vi "FGGA Linelock Settings Procedures.vi"() -> ()   [LabVIEW 2014]
panel:
  out "CO preflight Des 4":string="This issue can be fixed without opening the instrument. However, it may take a little bit of trial an error to get the exact adjustment. The goal is to bring the laser peaks back to their “normal” positions.\n\n1) On the instrument interface, click the Setup button in right hand corner of dashboard\n2) Click Service\n3) In the dialog window, enter ICOService (case sensitive)\n4) Click OK\n5) When the desktop appears, right click anywhere on the desktop\n6) Highlight Open New Window\n7) Click Up twice\n8) Scroll down to folder titled usr\n9) Double click usr\n10)Double click folder titled icos\n11)Double click folder titled conf\n12)Double Click folder titled fgga_ini\n13) If it is the Methane/H2O laser that needs adjusting, right click on filename linelock_0.ini. If it is the CO2 laser that needs adjusting, right click on filename linelock_1.ini.\n14)Highlight Open with…\n15) Click on gedit\n16) Increase the value of V0 by 0.1. For example, if V0 = -3.518, change it to -3.418.\n17)Hit CTRL-S to save changes\n18) Close all open windows\n19)Move the mouse to the top of display screen\n20) When a menu bar appears, click the LGR icon to restart instrument\n21)Go to the spectra screen again to check the new location of the spectral peaks.\n22) Repeat the procedure until the peak s are in the correct position. If the peaks move in the wrong direction, subtract in 0.1 increments instead of adding. If the peaks have moved far, it may take two three iterations to move them to the correct position. Smaller increments can also be used to shift the peaks smaller amounts.\n\n\n\n\n\n\n\n\n\n\n\n\n\n\n\n\n\n\n\n\n\n\n\n\n\n\n\n\n\n\n\n\n\n\n\n\n\n\n\n\n\n\n\n\n\n\n\n\n\n\n\n\n\n\n\n\n\n\n\n"
  out "CO preflight Des 3":string="The picture below is one that was sent to us by one of our customers in which the CO2 laser had shifted so much to the right that most of the peak is off the screen (from 0 to >10). The measured value of CO2 in this situation was -1.0000 which is a classic symptom of this issue.\n\n\n\n\n\n\n\n\n\n\n\n\n\n\n\n\n\n\n\n\n\n\n\n\n\n\n\n\n\n\n\n\n\n\n\n\n\n\n\n\n\n\n\n\n\n\n\n\n\n\n\n\n\n\n\n\n\n\n\n"
  out "CO preflight Des 2":string="The figure below show abnormal spectra in which the laser peaks have shifted to the left so that they need adjusting (big peak now at about -16).\n\n\n\n\n\n\n\n\n\n\n\n\n\n\n\n\n\n\n\n\n\n\n\n\n\n\n\n\n\n\n\n\n\n\n\n\n\n\n\n\n\n\n\n\n\n\n\n\n\n\n\n\n\n\n\n\n\n\n\n\n"
  out "CO preflight Des 1":string="Procedure for Change Linelock Settings\n\nThe goal of this procedure is to adjust the linelock voltage to bring the laser absorption peaks to the expected position in the absorption spectrum so that the instrument can measure properly.\nAs instrument lasers age, they may shift frequency. This is normal. The instrument is programmed to still make accurate measurements even when the lasers have shifted a bit, but if the situation continues, the instrument will not be able to compensate and the measurements will be affected. The status of the laser shift can be observed by reviewing the lower graph in the spectrum screen. There are two lasers in the instrument. The spectra for each laser can be toggled by selecting the appropriate species in the lower right of the screen.\nThe figure below shows normal spectra for the laser the measures methane and water vapor (big peak at about -12):\n\n\n\n\n\n\n\n\n\n\n\n\n\n\n\n\n\n\n\n\n\n\n\n\n\n\n\n\n\n"
  in  "Exit":bool
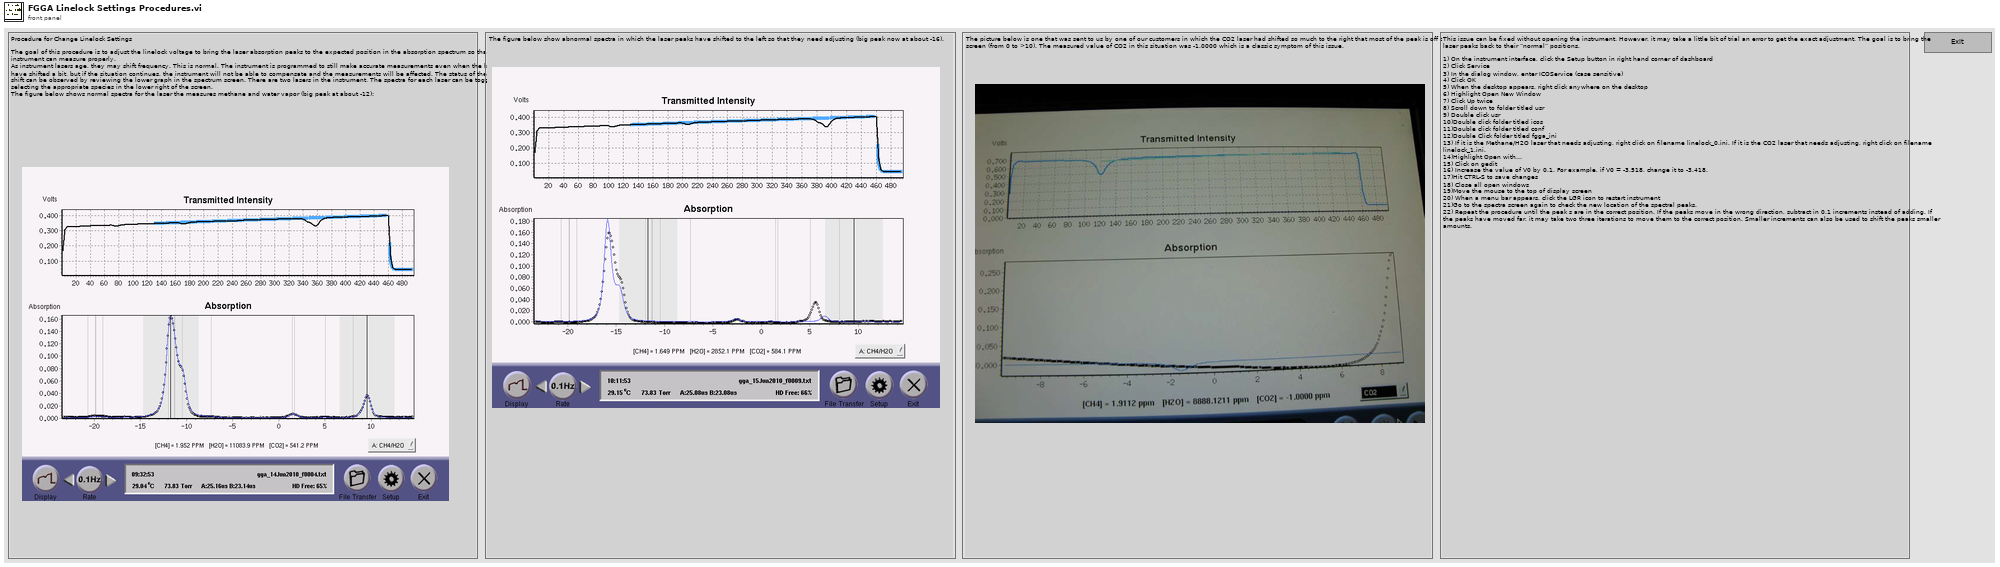
[diagram p1: front panel]
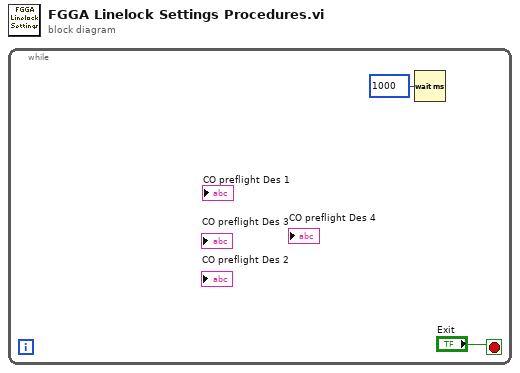
[diagram p0: block diagram]
diagram:
  n1 = while {
    stop <- "Exit" stop-if-true
    n2 = Wait (ms)(milliseconds to wait=u32 1000) -> ()  [unwired: 1 out]
  }
